vi "Read Y.vi"(8 "error in (no error)":errorcluster, 11 "JumpAbs in":refnum<class "MarkRel.lvclass">) -> (0 "error out":errorcluster, 2 "Y":dbl, 3 "JumpAbs out":refnum<class "MarkRel.lvclass">)   [LabVIEW 2013, in "MaterialCharacterization.lvlib" / "MarkRel.lvclass"]
uses:
  MarkRel.lvclass
  MarkRel.lvclass/MarkRel.ctl
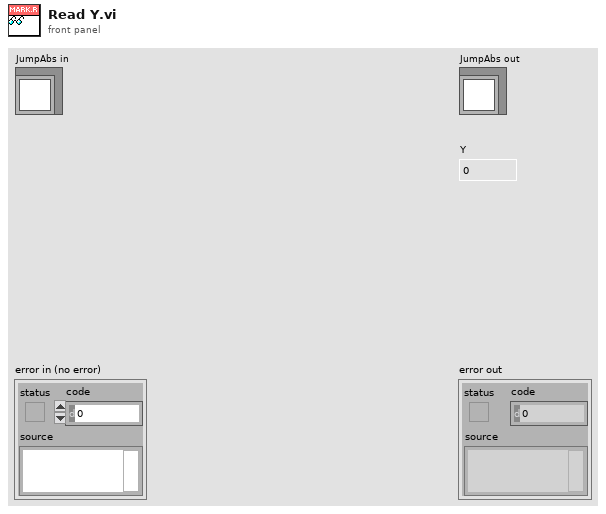
[diagram p1: front panel]
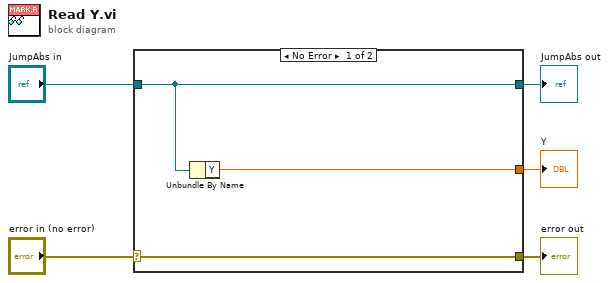
[diagram p0: block diagram]
diagram:
  n1 = case shown="No Error" "error in (no error)" {
    selector: "error in (no error)" -> [w8 w9]
    tunnel: [w8 w9] -> w4
    tunnel: [w7 w10] -> w2
    tunnel: "JumpAbs in" -> [w7 w10]
    tunnel: [w6 _] -> w1
    frame No Error {
      n2 = Unbundle By Name(w7) -> ("Y"=w6:dbl)
    }
    frame Error {
    }
  }
  "error out" <- w4
  "JumpAbs out" <- w2
  "Y" <- w1
